vi "Read All Strings.vi"(8 "error in (no error)":errorcluster, 11 "STEP in":T1) -> (0 "error out":errorcluster, 1 "All Strings":string[](array[string]), 3 "STEP out":T1)   [LabVIEW 2014, in "SeqLoop.lvlib"]
uses:
  TypeDefs/STEP.ctl
  TypeDefs/LogicParsedExpression.ctl
  Mimico Display/TypeDefs/Mimic Data.ctl
  Mimico Display/TypeDefs/BG Image.ctl
  Mimico Display/TypeDefs/mObject.ctl
  SeqLoop.lvlib
  Mimico Display/Mimico Display.lvlib
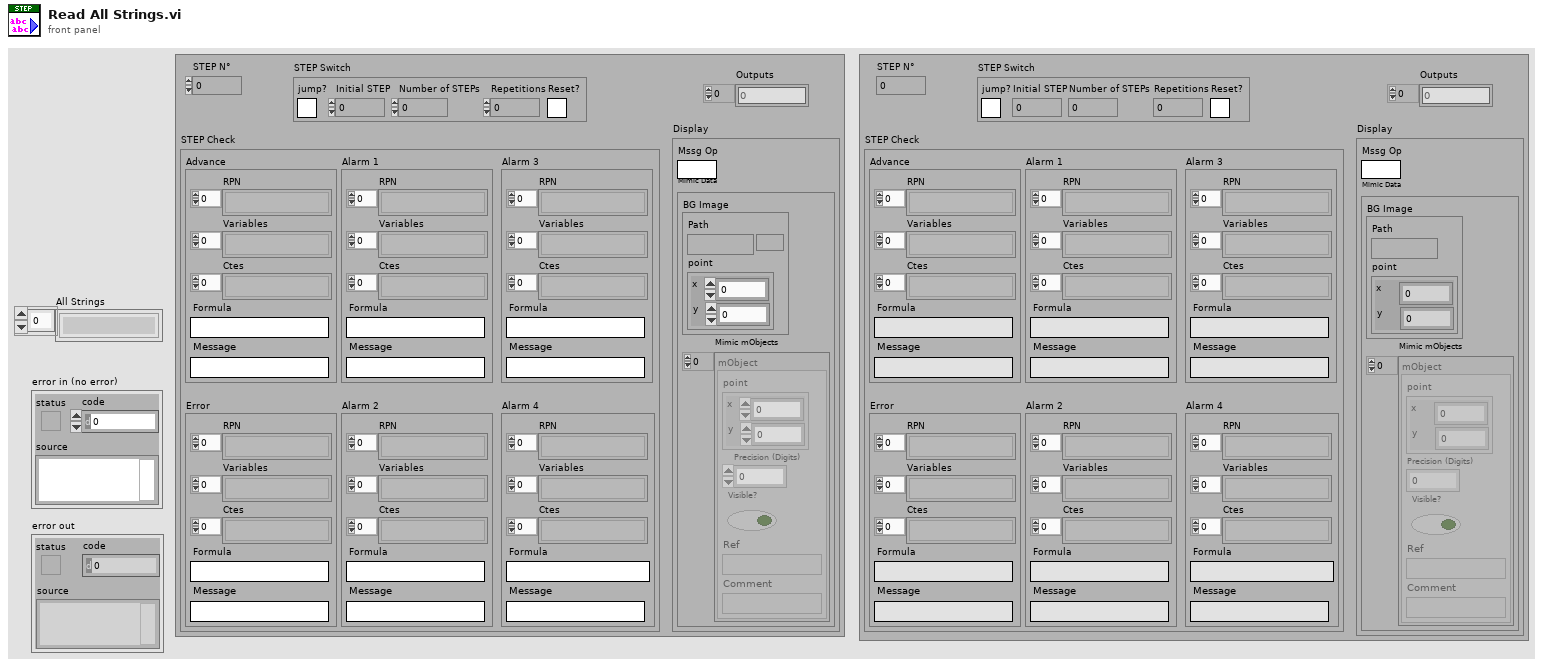
[diagram p1: front panel]
types:
  T1 = typedef "SeqLoop.lvlib/STEP.ctl" = cluster{"STEP N°":u32, "STEP Switch":cluster{"jump?":bool, "Initial STEP":u32, "Number of STEPs":u32, "Repetitions":u32, "Reset?":bool}, "Outputs":i32[], "STEP Check":cluster{"Advance":T2, "Error ":T2, "Alarm 1":T2, "Alarm 2":T2, "Alarm 3":T2, "Alarm 4":T2}, "Display":cluster{"Mssg Op":string, "Mimic Data":T3}}
  T2 = typedef "SeqLoop.lvlib/LogicParsedExpression.ctl" = cluster{"RPN ":string[], "Variables":string[], "Ctes":string[], "Formula":string, "Message":string}
  T3 = typedef "SeqLoop.lvlib/Mimico Display.lvlib/Mimic Data.ctl" = cluster{"BG Image":T4, "Mimic mObjects":T5[]}
  T4 = typedef "SeqLoop.lvlib/Mimico Display.lvlib/BG Image.ctl" = cluster{"Path":path, "point":cluster{"x":i16, "y":i16}}
  T5 = typedef "SeqLoop.lvlib/Mimico Display.lvlib/mObject.ctl" = cluster{"point":cluster{"x":i16, "y":i16}, "Precision (Digits)":i32, "Visible?":bool, "Ref":string, "Comment":string}
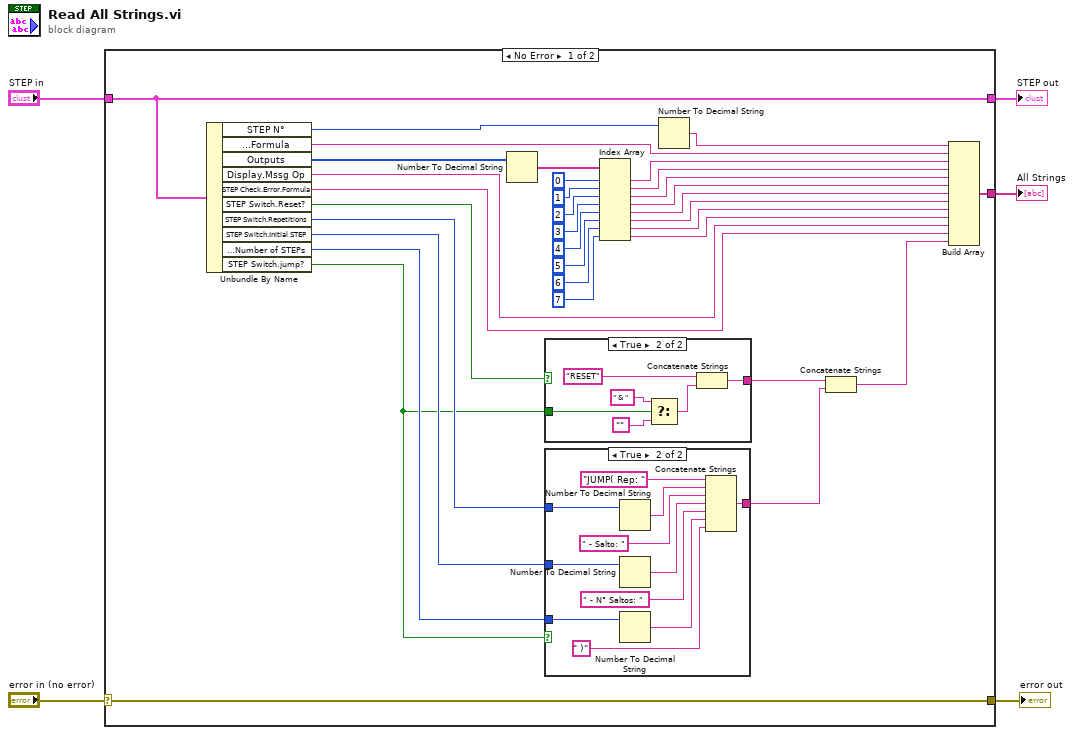
[diagram p0: block diagram]
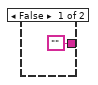
[diagram p2: hidden frame]
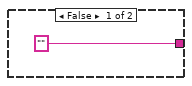
[diagram p3: hidden frame]
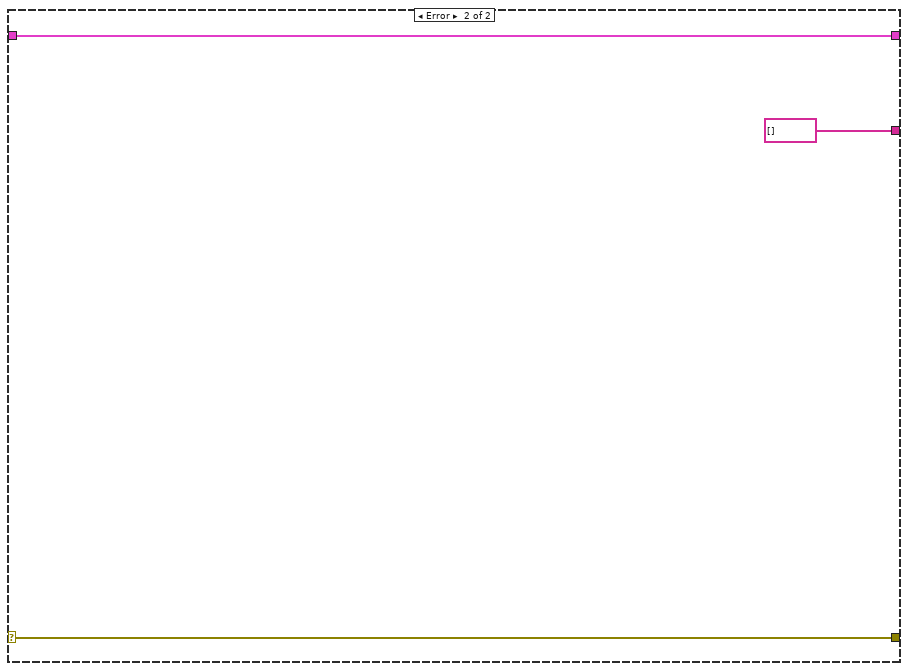
[diagram p4: hidden frame]
diagram:
  n1 = case shown="No Error" "error in (no error)" {
    selector: "error in (no error)" -> [w39 w61]
    tunnel: [w39 w61] -> w4
    tunnel: "STEP in" -> [w6 w59]
    tunnel: [w15 string[] []] -> w3
    tunnel: [w6 w59] -> w2
    frame No Error {
      n2 = Unbundle By Name(w6) -> ("STEP N°"=w27:u32, "STEP Check.Advance.Formula"=w28:string, "Outputs"=w25:i32[], "Display.Mssg Op"=w37:string, "STEP Check.Error.Formula"=w38:string, "STEP Switch.Reset?"=w11:bool, "STEP Switch.Repetitions"=w10:u32, "STEP Switch.Initial STEP"=w9:u32, "STEP Switch.Number of STEPs"=w8:u32, "STEP Switch.jump?"=w7:bool)
      n3 = Number To Decimal String(number=w25) -> (decimal integer string=w24:string[])  [unwired: 1 in]
      n4 = case shown="True" w11 {
        tunnel: ["" w56] -> w14
        tunnel: w7 -> [_ w58]
        frame False {
        }
        frame True {
          (unwired) "RESET"
          n5 = Select(t=" & ", s=w58, f="") -> (s? t:f=w55:string)
          n6 = Concatenate Strings("RESET", w55) -> (w56:string)
        }
      }
      n7 = case shown="True" w7 {
        tunnel: w10 -> [_ w51]
        tunnel: w9 -> [_ w50]
        tunnel: w8 -> [_ w49]
        tunnel: ["" w48] -> w13
        frame False {
        }
        frame True {
          n8 = Number To Decimal String(number=w51) -> (decimal integer string=w46:string)  [unwired: 1 in]
          n9 = Number To Decimal String(number=w50) -> (decimal integer string=w45:string)  [unwired: 1 in]
          n10 = Number To Decimal String(number=w49) -> (decimal integer string=w42:string)  [unwired: 1 in]
          n11 = Concatenate Strings("JUMP( Rep: " ("string"), w46, " - Salto: " ("string"), w45, " - N° Saltos: " ("string"), w42, " )" ("string")) -> (w48:string)
        }
      }
      n12 = Index Array(array=w24, index #1=0 ("index"), index #2=1 ("index 2"), index #3=2 ("index 3"), index #4=3 ("index 4"), index #5=4 ("index 5"), index #6=5 ("index 6"), index #7=6 ("index 7"), index #8=7 ("index 8")) -> (element #1=w23:string, element #2=w16:string, element #3=w17:string, element #4=w18:string, element #5=w19:string, element #6=w20:string, element #7=w21:string, element #8=w22:string)
      n13 = Number To Decimal String(number=w27) -> (decimal integer string=w26:string)  [unwired: 1 in]
      n14 = Concatenate Strings(w14, w13) -> (w12:string)
      n15 = Build Array(w26, w28, w23, w16, w17, w18, w19, w20, w21, w22, w37, w38, w12) -> (w15:string[])
    }
    frame Error {
    }
  }
  "error out" <- w4
  "All Strings" <- w3
  "STEP out" <- w2
